vi "CDS structure.vi"(11 "inReplace":variant) -> (3 "outReplace":variant)   [LabVIEW 2018]
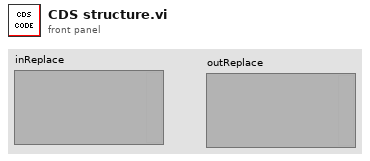
[diagram p1: front panel]
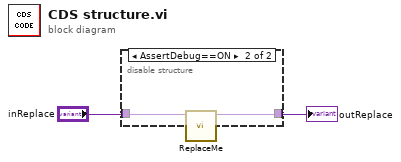
[diagram p0: block diagram]
diagram:
  n1 = disable-structure "AssertVI_CDS" shown="AssertDebug==ON" {
    disable-tunnel: [w3 w4] -> w2
    disable-tunnel: "inReplace" -> [w3 w5]
    frame condition #0 (active) {
    }
    frame condition #1 {
      # "Assert"
      n2 = call "ReplaceMe.vi"("In"=w5) -> ("Out"=w4:variant)  [unwired: 10 in]
    }
  }
  "outReplace" <- w2
